vi "Get-state-string.vi"(11 "States":T1) -> (3 "State string":string)   [LabVIEW 2013, in "SLMControl.lvlib" / "SC-UI.lvclass"]
uses:
  SC-UI.lvclass
  Main/Main-actions.ctl
  Main/SC-Main.lvclass
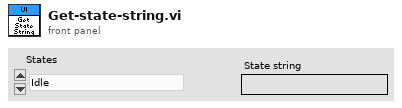
[diagram p1: front panel]
types:
  T1 = typedef "SLMControl.lvlib/SC-Main.lvclass/Main-actions.ctl" = enum16{"Idle", "Initialize", "Load configuration", "Save configuration", "Load lasing files", "Load deposition files", "Refresh files", "Clear files", "Open lasing file", "Activate", "Start", "Start deposition cycle", "Start lasing cycle", "Iterate", "Abort", "Stop", "Exit"}
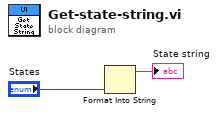
[diagram p0: block diagram]
diagram:
  n1 = Format Into String("States") -> (resulting string=→"State string":string)  [unwired: 3 in, 1 out]
